vi "Parse Digital Waveform.vi"(10 "Digital Wave":digitalwaveform(waveform)={"t0"=timestamp(0 s since 1904-01-01), "dt"=1.0, "Y"={"transitions"=[], "data"=[]}}) -> (1 "Y":digitaldata, 2 "dt":dbl, 4 "Boolean":bool=TRUE, 5 "t0":timestamp, 6 "attributes":variant)   [LabVIEW 2021]
uses:
  <vilib>/Waveform/DTblOps.llb/DTbl Digital to Boolean Array.vi
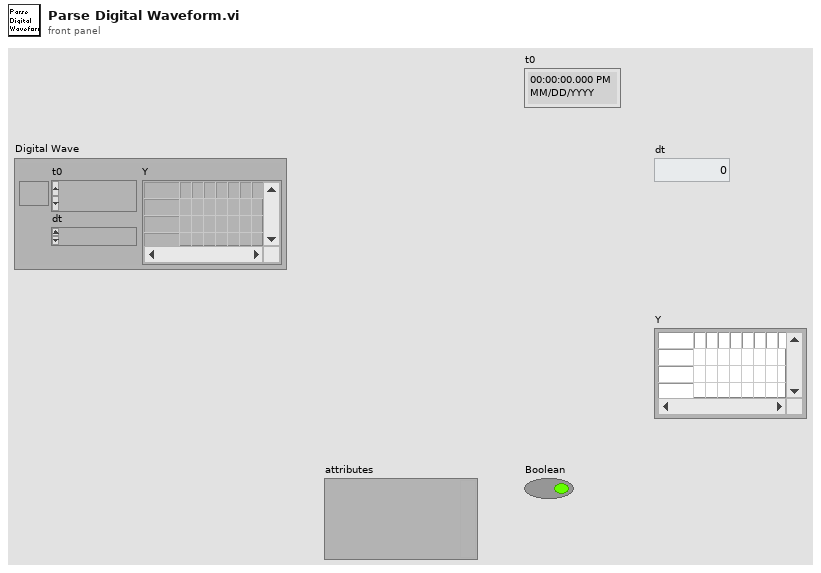
[diagram p1: front panel]
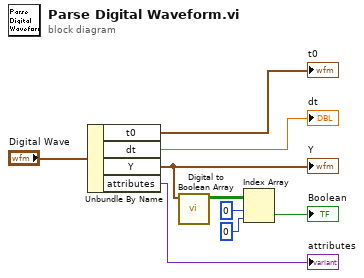
[diagram p0: block diagram]
diagram:
  n1 = Unbundle By Name("Digital Wave") -> ("t0"=→"t0":timestamp, "dt"=→"dt":dbl, "Y"=w8:digitaldata, "attributes"=→"attributes":variant)
  "Y" <- w8
  n2 = call-poly <vilib>:"Digital to Boolean Array.vi"("digital data"=w8) -> ("boolean array"=w7:bool[][])  [unwired: 9 in, 1 out]
  n3 = Index Array(array=w7, index (row)=0, index (col)=0 ("disabled index (col)")) -> (element=→"Boolean":bool)
